vi "Home_Ref_API.vi"(0 "DVR In":refnum<data-value>, 11 "Error In":errorcluster) -> (4 "DVR Out":refnum<data-value>, 6 "VI Ref":refnum<vi>, 8 "Home Ref":refnum<vi>, 15 "Error Out":errorcluster)   [LabVIEW 2020, in "Test.lvclass"]
doc: "Home Reference API"
uses:
  Test.lvclass
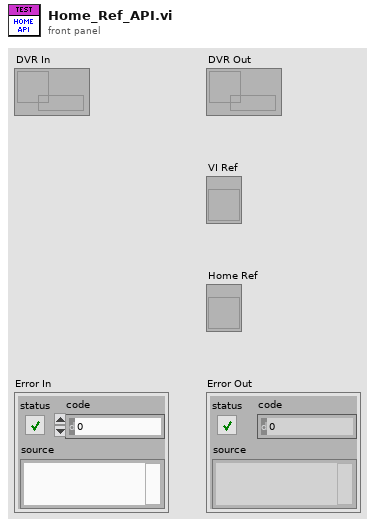
[diagram p1: front panel]
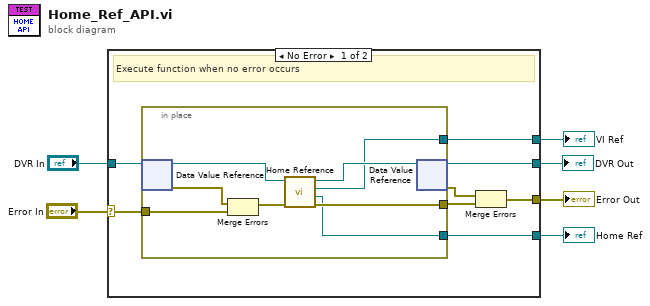
[diagram p0: block diagram]
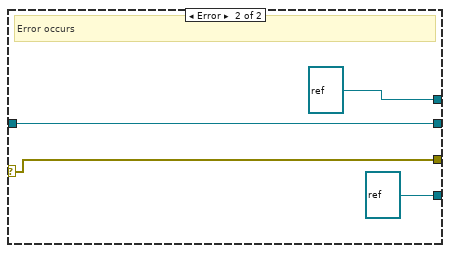
[diagram p2: hidden frame]
diagram:
  n1 = case shown="No Error" "Error In" {
    selector: "Error In" -> [w13 w26]
    tunnel: "DVR In" -> [w14 w25]
    tunnel: [w10 w26] -> w4
    tunnel: [w9 w25] -> w3
    tunnel: [w8 refnum<vi> refnum ("VI Ref")] -> w2
    tunnel: [w7 refnum<vi> refnum ("Home Ref")] -> w1
    frame No Error {
      # "Execute function when no error occurs"
      n2 = in-place {
        in-place-border: w13 -> [w21]
        in-place-border: [w17] -> w8
        in-place-border: [w16] -> w11
        in-place-border: [w15] -> w7
        n3 = in-place-dvr #1(w14) -> (w19:refnum<class "Test.lvclass">, w22:errorcluster)
        n4 = Merge Errors(w22, w21) -> (w20:errorcluster)
        n5 = call-dynamic "Home Reference.vi"("Error in"=w20, "Test in"=w19) -> ("Error out"=w16:errorcluster, "Home Ref"=w15:refnum<vi>, "VI Ref"=w17:refnum<vi>, "Test out"=w18:refnum<class "Test.lvclass">)  [unwired: 6 in]
        n6 = in-place-dvr #1(w18) -> (w9:refnum<data-value>, w12:errorcluster)
      }
      n7 = Merge Errors(w12, w11) -> (w10:errorcluster)
    }
    frame Error {
      # "Error occurs"
    }
  }
  "Error Out" <- w4
  "DVR Out" <- w3
  "VI Ref" <- w2
  "Home Ref" <- w1
